vi "FTW-MessagePayload-Decompose.vi"(0 "Message":T1) -> (2 "Sender Identity":string, 3 "Message Header":string, 4 "Message Body":string)   [LabVIEW 2013]
uses:
  FTW-MessagePayload.ctl
panel:
  # "Inputs"
  # "Outputs"
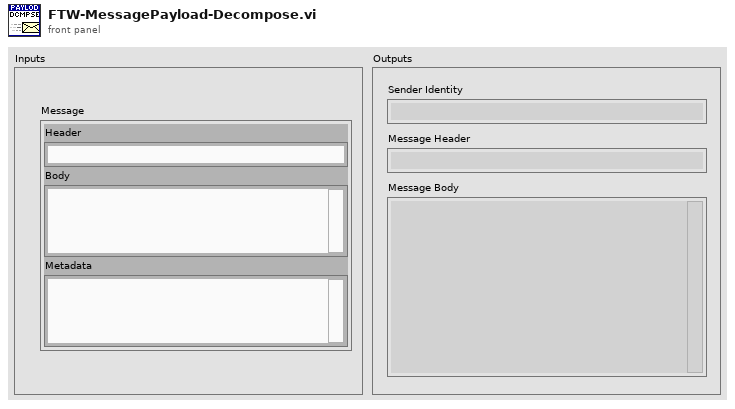
[diagram p1: front panel]
types:
  T1 = typedef "FTW-MessagePayload.ctl" = cluster{"Header":string, "Body":string, "Metadata":string}
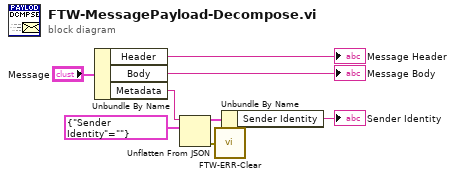
[diagram p0: block diagram]
diagram:
  n1 = Unbundle By Name("Message") -> ("Header"=→"Message Header":string, "Body"=→"Message Body":string, "Metadata"=w5:string)
  n2 = Unflatten From JSON(JSON string=w5, type and defaults=cluster{"Sender Identity":string} {"Sender Identity"=""}) -> (value=w2:cluster{"Sender Identity":string}, error out=w3:errorcluster)  [unwired: 5 in]
  n3 = call "FTW-ERR-Clear.vi"("error to snuff"=w3) -> ()  [unwired: 1 out]
  n4 = Unbundle By Name(w2) -> ("Sender Identity"=→"Sender Identity":string)
